vi "MU Update Mt Sync.vi"(8 "error in (no error)":errorcluster, 10 "MtAnalyzeResultHandle":T1, 11 "MuHandle":u64) -> (0 "error out":errorcluster, 3 "function return":u32)   [LabVIEW 2022 SP3, in "MU_3SL_interface.lvlib"]
uses:
  MU_3SL_interface.lvlib
  handles/mtSyncAnalyzeResultHandle.ctl
  lib/MU_3SL_interface_64.dll
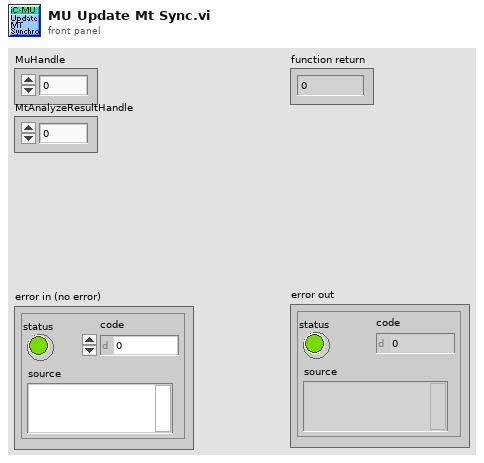
[diagram p1: front panel]
types:
  T1 = typedef "MU_3SL_interface.lvlib/mtSyncAnalyzeResultHandle.ctl" = u64
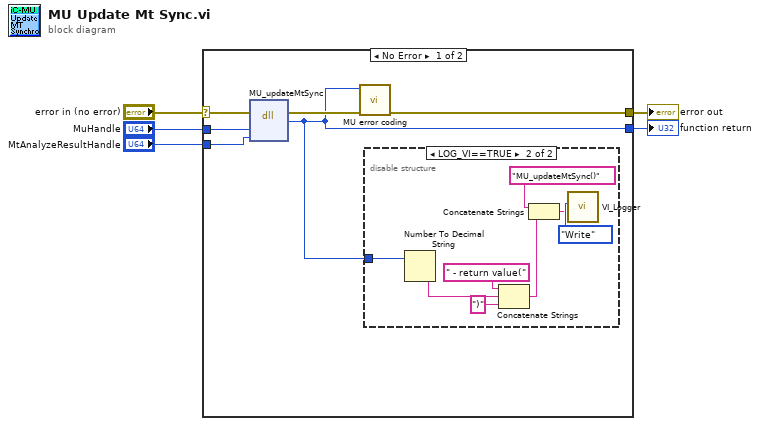
[diagram p0: block diagram]
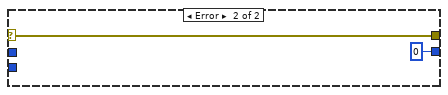
[diagram p3: hidden frame]
diagram:
  n1 = case shown="No Error" "error in (no error)" {
    selector: "error in (no error)" -> [w11 w21]
    tunnel: [w6 u32 0 ("function return")] -> w1
    tunnel: [w7 w21] -> w5
    tunnel: "MuHandle" -> [w10 _]
    tunnel: "MtAnalyzeResultHandle" -> [w9 _]
    frame No Error {
      n2 = dll-call lib="C:/Users/bes/AppData/Roaming/work/mu_9so/icsubmodules/soft_mu_3sl_master/lv_interface/lib/MU_3SL_interface**.*" fn="MU_updateMtSync"(error in=w11, "MuHandle"=w10, "MtAnalyzeResultHandle"=w9) -> (error out=w8:errorcluster, "function return"=w6:u32)  [unwired: 4 in, 1 out]
      n3 = call "MU error coding.vi"("error in (no error)"=w8, "function return in"=w6) -> ("error out"=w7:errorcluster)  [unwired: 9 in]
      n4 = disable-structure shown="LOG_VI==TRUE" {
        disable-tunnel: w6 -> [_ w13]
        frame condition #0 {
        }
        frame condition #1 (active) {
          n5 = Number To Decimal String(number=w13) -> (decimal integer string=w12:string)  [unwired: 1 in]
          n6 = Concatenate Strings(" - return value(" ("string"), w12, ")" ("string")) -> (w17:string)
          n7 = Concatenate Strings("MU_updateMtSync()" ("Info in"), w17) -> (w16:string)
          n8 = call "VI_Logger.vi"("Action (Read)"=enum16{"Write", "Read"}."Write", "Info in"=w16) -> ()  [unwired: 8 in, 2 out]
        }
      }
    }
    frame Error {
    }
  }
  "error out" <- w5
  "function return" <- w1
